vi "Close Instrument Sessions.vi"(0 "Scalar SG Si2250 Path Group in":refnum<class "SG SC2250 Path Group.lvclass">, 11 "error in (no error)":errorcluster) -> (4 "Scalar SG Si2250 Path Group out":refnum<class "SG SC2250 Path Group.lvclass">, 15 "error out":errorcluster)   [LabVIEW 2023, in "RFFixtureCharact.RFPM.lvlib" / "SG SC2250 Path Group.lvclass"]
uses:
  SG SC2250 Path Group.lvclass
  Instruments/Power Meter/Power Meter Factory/Power Meter Factory.lvclass
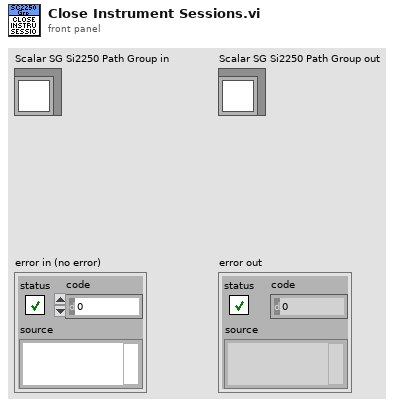
[diagram p1: front panel]
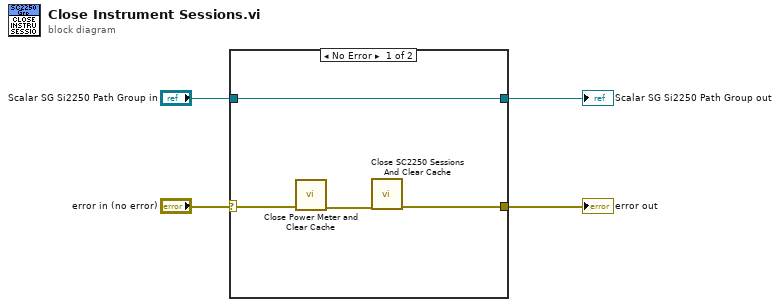
[diagram p0: block diagram]
diagram:
  n1 = case shown="No Error" "error in (no error)" {
    selector: "error in (no error)" -> [w5 w10]
    tunnel: "Scalar SG Si2250 Path Group in" -> [w8 w9]
    tunnel: [w8 w9] -> w2
    tunnel: [w7 w10] -> w1
    frame No Error {
      n2 = call "Close Power Meter and Clear Cache.vi"("error in (no error)"=w5) -> ("error out"=w6:errorcluster)  [unwired: 14 in]
      n3 = call "Close SC2250 Sessions And Clear Cache.vi"("error in (no error)"=w6) -> ("error out"=w7:errorcluster)  [unwired: 14 in]
    }
    frame Error {
    }
  }
  "error out" <- w1
  "Scalar SG Si2250 Path Group out" <- w2
